vi "Helper SubVI - Sine Curve Fitting Prepare.vi"(11 "signal in":waveform(dbl)) -> (3 "signal out":waveform(dbl))   [LabVIEW 2023]
doc: "Preprocesses a signal to form Gaussian pulses."
uses:
  <vilib>/Analysis/baseanly.llb/Mean (DBL).vi
  <vilib>/Analysis/NI_AALBase.lvlib
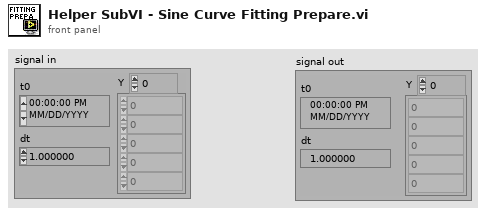
[diagram p1: front panel]
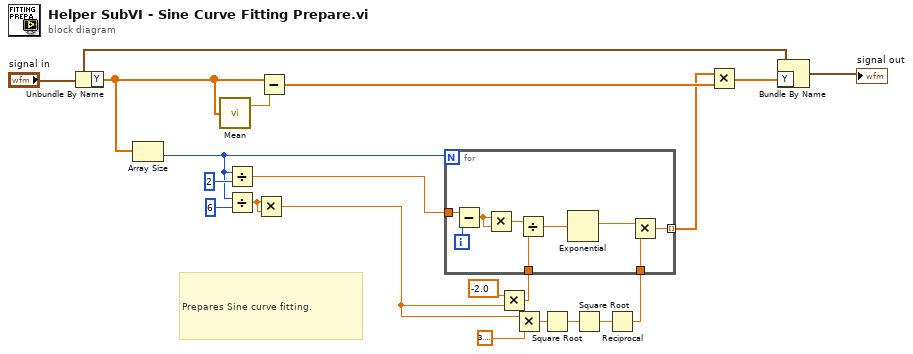
[diagram p0: block diagram]
diagram:
  # "Prepares Sine curve fitting."
  n1 = Unbundle By Name("signal in") -> ("Y"=w13:dbl[])
  n2 = Array Size(array=w13) -> (size(s)=w4:i32)
  n3 = call-poly <vilib>:"Mean.vi"("X"=w13) -> ("mean"=w20:dbl)  [unwired: 1 out]
  n4 = Divide(x=w4, y=2) -> (x/y=w3:dbl)
  n5 = Divide(x=w4, y=6) -> (x/y=w15:dbl)
  n6 = Multiply(x=w15, y=w15) -> (x*y=w2:dbl)
  n7 = Subtract(x=w13, y=w20) -> (x-y=w19:dbl[])
  n8 = Multiply(x=-2.0, y=w2) -> (x*y=w6:dbl)
  n9 = Multiply(x=w2, y=3.141592653589793) -> (x*y=w10:dbl)
  n10 = Square Root(x=w10) -> (sqrt(x)=w9:dbl)
  n11 = Square Root(x=w9) -> (sqrt(x)=w8:dbl)
  n12 = Reciprocal(x=w8) -> (1/x=w5:dbl)
  n13 = for {
    N: w4 -> [_]
    tunnel: w3 -> [w29]
    tunnel: w6 -> [w25]
    tunnel: w5 -> [w23]
    tunnel: [w22] -> w1 mode=indexing
    i -> [w28]
    n14 = Subtract(x=w29, y=w28) -> (x-y=w27:dbl)
    n15 = Multiply(x=w27, y=w27) -> (x*y=w26:dbl)
    n16 = Divide(x=w26, y=w25) -> (x/y=w21:dbl)
    n17 = Exponential(1:w21) -> (0:w24:dbl)
    n18 = Multiply(x=w24, y=w23) -> (x*y=w22:dbl)
  }
  n19 = Multiply(x=w1, y=w19) -> (x*y=w14:dbl[])
  n20 = Bundle By Name(cluster="signal in", "Y"=w14) -> (→"signal out":waveform(dbl))
